vi "Read Alarms Event Response.vi"(8 "error in (no error)":errorcluster, 11 "Alarms in":refnum<class "HK Alarms.lvclass">) -> (0 "error out":errorcluster, 2 "Alarms":T1[](array[typedef]), 3 "Alarms out":refnum<class "HK Alarms.lvclass">)   [LabVIEW 2024, in "HK Alarms.lvclass"]
uses:
  HK Alarms.lvclass
  HK Channel Settings Alarms.ctl
  HK Alarm enum Action.ctl
  HK Alarms.lvclass/HK Alarms.ctl
  HK Item/HK Item.lvclass
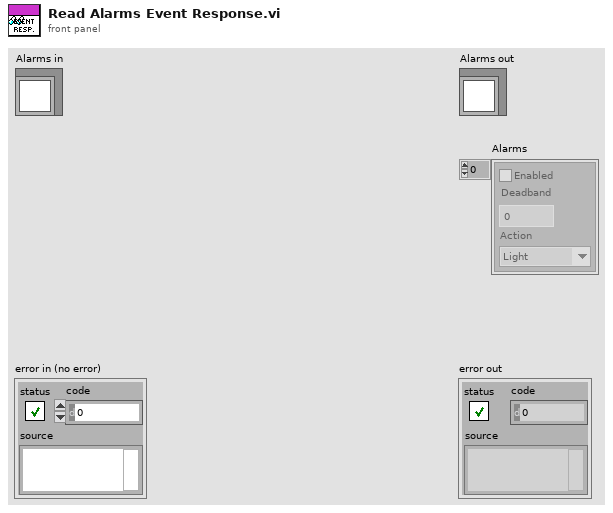
[diagram p1: front panel]
types:
  T1 = typedef "HK Item.lvclass/HK Channel Settings Alarms.ctl" = cluster{"Enabled":bool, "Deadband":i32, "Action":T2}
  T2 = typedef "HK Item.lvclass/HK Alarm enum Action.ctl" = enum16{"Light", "Message", "Safe"}
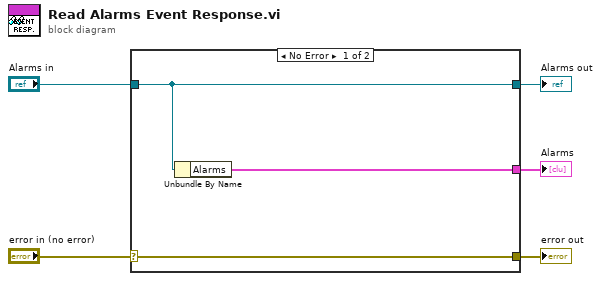
[diagram p0: block diagram]
diagram:
  n1 = case shown="No Error" "error in (no error)" {
    selector: "error in (no error)" -> [w8 w9]
    tunnel: [w8 w9] -> w4
    tunnel: [w7 w10] -> w2
    tunnel: "Alarms in" -> [w7 w10]
    tunnel: [w6 _] -> w1
    frame No Error {
      n2 = Unbundle By Name(w7) -> ("Alarms"=w6:T1[])
    }
    frame Error {
    }
  }
  "error out" <- w4
  "Alarms out" <- w2
  "Alarms" <- w1
